vi "parse_cmd.vi"(8 "error in (no error)":errorcluster, 11 "CMD In":string=":CALCulate:ACPower:LIMit:STATe OFF|ON|0|1") -> (0 "error out":errorcluster, 1 "Polished CMD":string, 2 "CMD Parameters":T1, 3 "CMD Out":string, 5 "Parsing Successful?":bool)   [LabVIEW 2018]
uses:
  TypeDefinitions/auto_extracted_control_specs.ctl
  TypeDefinitions/auto_extracted_control_spec.ctl
  Gtor/Mth/GenVI/Intf/GenStdVI/Mth/GenOneStdVI/TypeDefinitions/control_data_type.ctl
  Gtor/Mth/GenVI/Intf/GenStdVI/Mth/GenOneStdVI/TypeDefinitions/control_class.ctl
  Gtor/Mth/GenVI/Intf/GenStdVI/Mth/GenOneStdVI/TypeDefinitions/ring_string_and_value.ctl
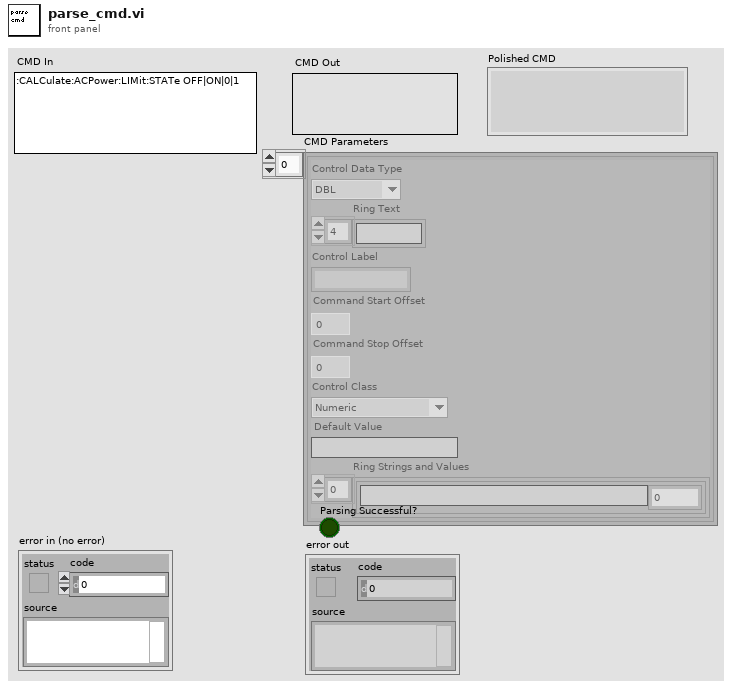
[diagram p1: front panel]
types:
  T1 = typedef "auto_extracted_control_specs.ctl" = T2[]
  T2 = typedef "auto_extracted_control_spec.ctl" = cluster{"Control Data Type":T3, "Ring Text":string[], "Control Label":string, "Command Start Offset":i32, "Command Stop Offset":i32, "Control Class":T4, "Default Value":string, "Ring Strings and Values":T5[]}
  T3 = typedef "control_data_type.ctl" = enum16{"DBL", "I32", "Boolean", "String", "U16", "U32", "EXT", "SGL", "I16", "U8", "I8", "I64", "U64", "Waveform", "Reference", "Variant", "Cluster"}
  T4 = typedef "control_class.ctl" = enum16{"Numeric", "Vertical Slide Switch", "Text Ring", "String", "Array", "VISAName", "WaveformGraph", "Cluster"}
  T5 = typedef "ring_string_and_value.ctl" = cluster{"String":string, "Value":dbl}
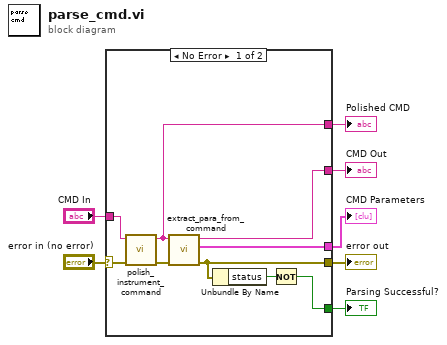
[diagram p0: block diagram]
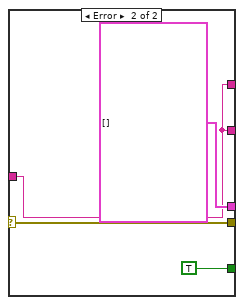
[diagram p2: hidden frame]
diagram:
  n1 = case shown="No Error" "error in (no error)" {
    selector: "error in (no error)" -> [w16 w20]
    tunnel: [w10 w20] -> w6
    tunnel: [w12 w18] -> w5
    tunnel: "CMD In" -> [w14 w18]
    tunnel: [w13 T1 [] ("Auto Extracted Contol Specs")] -> w3
    tunnel: [w11 w18] -> w2
    tunnel: [w8 TRUE] -> w1
    frame No Error {
      n2 = call "polish_instrument_command.vi"("error in (no error)"=w16, "Instrument Command In"=w14) -> ("error out"=w15:errorcluster, "Instrument Command Out"=w11:string)  [unwired: 8 out]
      n3 = call "extract_para_from_command.vi"("error in (no error)"=w15, "Instrument Command In"=w11) -> ("error out"=w10:errorcluster, "Auto Extracted Contol Specs"=w13:T1, "Instrument Command In Out"=w12:string)  [unwired: 7 out]
      n4 = Unbundle By Name(w10) -> ("status"=w9:bool)
      n5 = Not(x=w9) -> (.not. x?=w8:bool)
    }
    frame Error {
    }
  }
  "CMD Out" <- w5
  "error out" <- w6
  "CMD Parameters" <- w3
  "Polished CMD" <- w2
  "Parsing Successful?" <- w1
